vi "set pockels cell.vi"(8 "error in (no error)":errorcluster, 11 "Waveform in":refnum<class "Waveform.lvclass">) -> (0 "error out":errorcluster, 3 "Waveform out":refnum<class "Waveform.lvclass">)   [LabVIEW 2012, in "Waveform.lvclass"]
uses:
  Waveform.lvclass
  Waveform.lvclass/Waveform.ctl
  <vilib>/measure/NI_MABase.lvlib
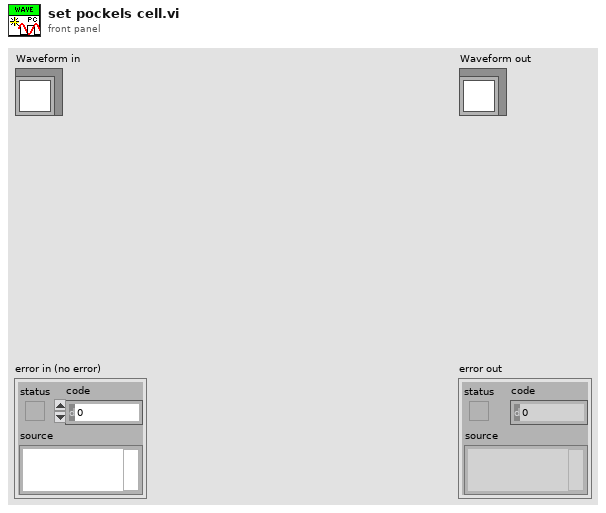
[diagram p1: front panel]
types:
  T1 = typedef "PC_wavelength.ctl" = dbl
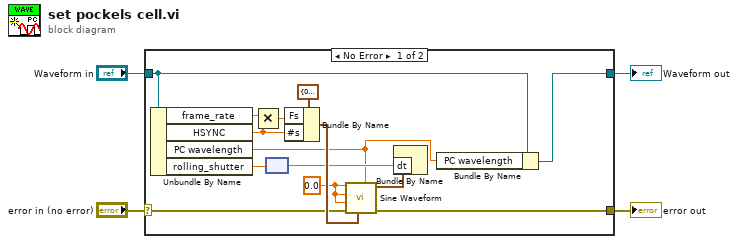
[diagram p0: block diagram]
diagram:
  n1 = case shown="No Error" "error in (no error)" {
    selector: "error in (no error)" -> [w13 w20]
    tunnel: [w12 w20] -> w3
    tunnel: [w6 w19] -> w1
    tunnel: "Waveform in" -> [w7 w19]
    frame No Error {
      w11 = 0.0
      n2 = Unbundle By Name(w7) -> ("frame_rate"=w16:dbl, "HSYNC"=w17:dbl, "PC wavelength"=w5:T1, "rolling_shutter"=w10:dbl[unit])
      n3 = Multiply(x=w16, y=w17) -> (x*y=w15:dbl)
      n4 = node(w10) -> (w9:dbl)
      n5 = Bundle By Name(cluster=cluster{"Fs":dbl, "#s":dbl} {"Fs"=0.0, "#s"=0.0} ("settings.Pockels Cell.sampling info"), "Fs"=w15, "#s"=w17) -> (w14:cluster{"Fs":dbl, "#s":dbl})
      n6 = call <vilib>:"Sine Waveform.vi"("offset"=w5, "sampling info"=w14, "error in (no error)"=w13, "phase"=w11, "amplitude"=w11, "frequency"=w11) -> ("error out"=w12:errorcluster, "signal out"=w8:waveform(dbl))  [unwired: 4 in]
      n7 = Bundle By Name(cluster=w8, "dt"=w9) -> ()  [unwired: 1 out]
      n8 = Bundle By Name(cluster=w7, "PC wavelength"=w5) -> (w6:refnum<class "Waveform.lvclass">)
    }
    frame Error {
    }
  }
  "error out" <- w3
  "Waveform out" <- w1
